vi "trajectory_new_code.vi"() -> ()   [LabVIEW 2019]
uses:
  <vilib>/FPGAPlugInAG/sbRIO-9629/niLvFpga_Open_sbRIO-9629.vi
  <vilib>/rvi/interface/common/dynamic/niFpgaDynamicAddResources.vi
  <vilib>/Utility/error.llb/Error Cluster From Error Code.vi
  <vilib>/rvi/errors/niLvFpgaAdjustHostInterfaceError.vi
  <vilib>/FPGAPlugInAG/Dynamic/niLvFpga_Close_Dynamic.vi
  <vilib>/rvi/interface/nirviOpenFPGA/nirviOpenFPGA.xnode
  FPGA Bitfiles/fcmsinglesection_FPGATarget_CloseLoopMotorTu_eGt+d+EV+VE.lvbitx
  Close_Loop_Motor_Tune.vi
  <vilib>/rvi/interface/nirviReadWriteControl/nirviReadWriteControl.xnode
  <vilib>/rvi/interface/nirviCloseFPGA/nirviCloseFPGA.xnode
  NiFpgaLv.dll
  <vilib>/rvi/interface/Simulation/niFpgaSimulationCallBeginRW.vi
panel:
  out "L_v":dbl
  out "alpha":dbl
  out "logical AND":bool
  in  "Lower limit":dbl[](array[numeric])
  in  "Upper limit":dbl[](array[numeric])
  in  "Kp":dbl[](array[numeric])
  out "Desired Tip Position":dbl[](array[numeric])
  in  "omega":dbl
  in  "r":dbl
  out "Error":dbl[](array[numeric])
  out "data out":string
  out "Current Tip Position":dbl[](array[numeric])
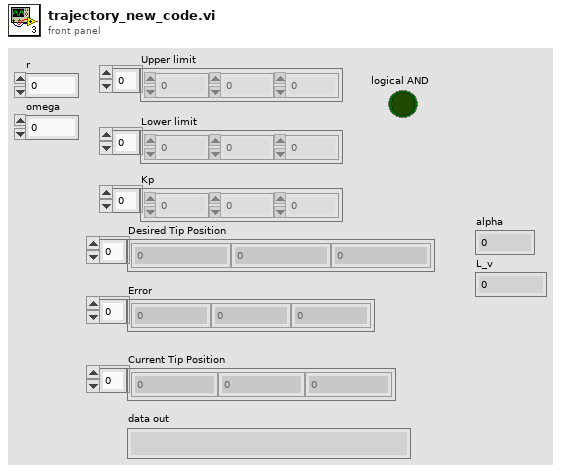
[diagram p1: front panel]
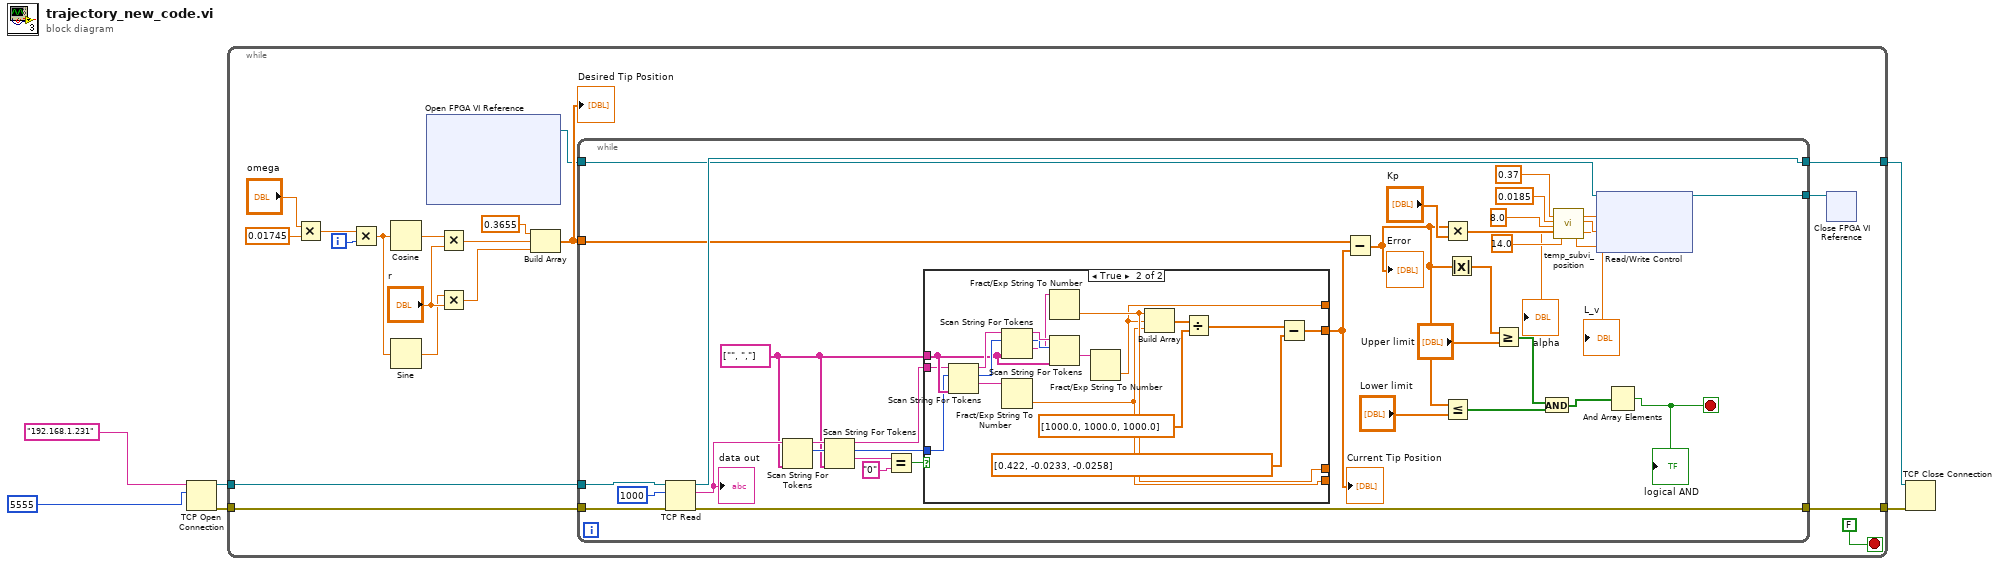
[diagram p0: block diagram]
diagram:
  n1 = TCP Open Connection(address="192.168.1.231", remote port or service name=u16 5555) -> (connection ID=w3:refnum<k5>, error out=w4:errorcluster)  [unwired: 3 in]
  n2 = while {
    tunnel: w4 -> [w24]
    tunnel: w3 -> [w23]
    tunnel: [w22] -> w2
    tunnel: [w21] -> w1
    i -> [w16]
    stop <- FALSE stop-if-true
    n3 = Multiply(x="omega", y=0.01745) -> (x*y=w17:dbl)
    n4 = Multiply(x=w17, y=w16) -> (x*y=w12:dbl)
    n5 = Cosine(x=w12) -> (cos(x)=w15:dbl)
    n6 = Sine(x=w12) -> (sin(x)=w11:dbl)
    n7 = xnode "Open FPGA VI Reference"() -> ("FPGA VI Reference Out"=w8:refnum<k20>)  [unwired: 2 in, 1 out]
    n8 = Multiply(x=w15, y="r") -> (x*y=w14:dbl)
    n9 = Multiply(x=w11, y="r") -> (x*y=w10:dbl)
    n10 = Build Array(0.3655 ("element"), w14, w10) -> (w9:dbl[])
    "Desired Tip Position" <- w9
    n11 = while {
      tunnel: [w52] -> w22
      tunnel: [w51] -> w21
      tunnel: w24 -> [w50]
      tunnel: w23 -> [w49]
      tunnel: w9 -> [w47]
      tunnel: w8 -> [w42]
      tunnel: [w41] -> w7
      stop <- w28 stop-if-true
      w55 = string[] ["", ","] ("delimiters (\\s,\\t,\\r,\\n)")
      n12 = TCP Read(connection ID=w49, bytes to read=1000, error in (no error)=w50) -> (connection ID out=w51:refnum<k5>, data out=w57:string, error out=w52:errorcluster)  [unwired: 2 in]
      "data out" <- w57
      n13 = Scan String For Tokens(6:w55, 9:w57) -> (2:w59:i32, 3:w60:string)  [unwired: 4 in, 2 out]
      n14 = Scan String For Tokens(6:w55, 8:w59, 9:w60) -> (1:w61:string, 2:w54:i32, 3:w53:string)  [unwired: 3 in, 1 out]
      n15 = Equal?(x=w61, y="0") -> (x = y?=w56:bool)
      n16 = case shown="True" w56 {
        tunnel: [_ w69] -> _
        tunnel: [_ w68] -> _
        tunnel: [_ w67] -> _
        tunnel: w55 -> [_ w66]
        tunnel: w54 -> [_ w65]
        tunnel: w53 -> [_ w64]
        tunnel: [_ w63] -> w48
        frame False {
        }
        frame True {
          n17 = Scan String For Tokens(6:w66, 8:w65, 9:w64) -> (1:w76:string, 2:w78:i32, 3:w80:string)  [unwired: 3 in, 1 out]
          n18 = Scan String For Tokens(6:w66, 8:w78, 9:w80) -> (1:w75:string, 2:w77:i32, 3:w79:string)  [unwired: 3 in, 1 out]
          n19 = Fract/Exp String To Number(string=w76) -> (number=w67:dbl)  [unwired: 3 in, 1 out]
          n20 = Fract/Exp String To Number(string=w75) -> (number=w69:dbl)  [unwired: 3 in, 1 out]
          n21 = Scan String For Tokens(6:w66, 8:w77, 9:w79) -> (1:w74:string)  [unwired: 3 in, 3 out]
          n22 = Fract/Exp String To Number(string=w74) -> (number=w68:dbl)  [unwired: 3 in, 1 out]
          n23 = Build Array(w69, w68, w67) -> (w73:dbl[])
          n24 = Divide(x=w73, y=dbl[] [1000.0, 1000.0, 1000.0]) -> (x/y=w71:dbl[])
          n25 = Subtract(x=w71, y=dbl[] [0.422, -0.0233, -0.0258]) -> (x-y=w63:dbl[])
        }
      }
      "Current Tip Position" <- w48
      n26 = Subtract(x=w47, y=w48) -> (x-y=w30:dbl[])
      "Error" <- w30
      n27 = Multiply(x=w30, y="Kp") -> (x*y=w36:dbl[])
      n28 = Less Or Equal?(x=w30, y="Lower limit") -> (x <= y?=w31:bool[])
      n29 = Absolute Value(x=w30) -> (abs(x)=w33:dbl[])
      n30 = Greater Or Equal?(x=w33, y="Upper limit") -> (x >= y?=w32:bool[])
      n31 = And(x=w32, y=w31) -> (x .and. y?=w29:bool[])
      n32 = call "temp_subvi_position.vi"("Length of the FCM (m)"=0.37, "Radius of disk (m)"=0.0185, "Number of Disks"=8.0, "Tip position"=w36, "Radius of pulley (mm)"=14.0) -> ("alpha"=→"alpha":dbl, "L_v"=→"L_v":dbl, "Theta 3"=w38:dbl, "Theta 1"=w40:dbl, "Theta 2"=w39:dbl)  [unwired: 4 in, 6 out]
      n33 = xnode "Read/Write Control"("FPGA VI Reference In"=w42, "desired angle"=w40, "desired angle 2"=w39, "desired angle 3"=w38) -> ("FPGA VI Reference Out"=w41:refnum<k20>)  [unwired: 1 in, 1 out]
      n34 = And Array Elements(Boolean array=w29) -> (logical AND=w28:bool)
      "logical AND" <- w28
    }
    n35 = xnode "Close FPGA VI Reference"("FPGA VI Reference In"=w7) -> ()  [unwired: 1 in, 1 out]
  }
  n36 = TCP Close Connection(connection ID=w1, error in (no error)=w2) -> ()  [unwired: 1 in, 2 out]
